vi "stiffnessChartView.vi"(10 "UserEvents in":refnum<class "UserEvents.lvclass">) -> ()   [LabVIEW 2013]
uses:
  UserEvents/UserEvents.lvclass
  UserEvents/UserEvents.lvclass/UserEvents.ctl
  Typedefs/StateSelector.ctl
  Typedefs/M2AADTTypedefs.lvlib
panel:
  out "Stiffness":dbl[unit] min=-888.0 max=888.0 format="%.2f"
  out "Stiffness vs. Move Number":dbl(graph)
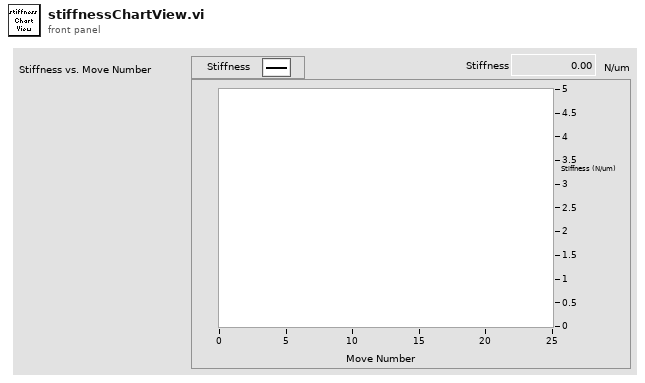
[diagram p1: front panel]
types:
  T1 = typedef "M2AADTTypedefs.lvlib/PubDataEvents.ctl" = cluster{"State":refnum<user-event>, "ErrorCode":refnum<user-event>, "OutputData":refnum<user-event>, "InputData":refnum<user-event>, "ControllerData":refnum<user-event>, "TestStatus":refnum<user-event>, "LogPath":refnum<user-event>, "StiffnessData":refnum<user-event>}
  T2 = cluster{"Event Registration Refnum":refnum<event-registration>, "Event Registration Refnum":refnum<event-registration>}
  T3 = typedef "M2AADTTypedefs.lvlib/StateSelector.ctl" = enum16{"EndingCycleState", "FaultState", "InteractiveMotionState", "MovingToNewForceState", "OffState", "PausingState", "StandbyState", "StoppedState"}
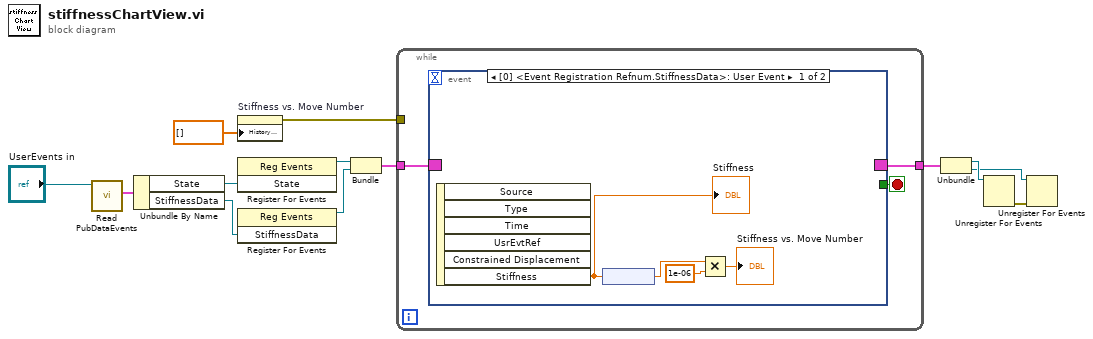
[diagram p0: block diagram]
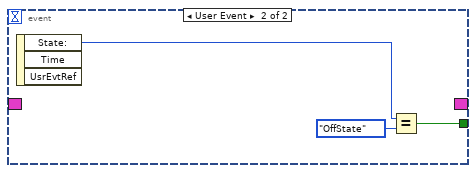
[diagram p2: hidden frame]
diagram:
  n1 = call "Read PubDataEvents.vi"("UserEvents in"="UserEvents in") -> ("PubDataEvents"=w13:T1)  [unwired: 9 in, 1 out]
  n2 = Unbundle By Name(w13) -> ("State"=w12:refnum<user-event>, "StiffnessData"=w3:refnum<user-event>)
  n3 = property on="Stiffness vs. Move Number" class="WFChart (strict)"("History Data"=dbl[] []) -> (error out=w4:errorcluster)  [unwired: 2 in, 1 out]
  n4 = register-events(w12) -> (reference out=w11:refnum<event-registration>)  [unwired: 2 in, 1 out]
  n5 = register-events(w3) -> (reference out=w2:refnum<event-registration>)  [unwired: 2 in, 1 out]
  n6 = Bundle("Event Registration Refnum"=w11, "Event Registration Refnum"=w2) -> (w9:T2)  [unwired: 1 in]
  n7 = while {
    tunnel: w9 -> [w16]
    tunnel: [w14] -> w8
    tunnel: w4 -> [_]
    stop <- w15 stop-if-true
    n8 = event shown="[0] <Event Registration Refnum.StiffnessData>: User Event" {
      selector: w16 -> [_ _]
      dyn-events: [_ _] -> w14
      timeout: _ -> [_ _]
      tunnel: [_ w22] -> w15
      event User Event {
        n9 = event-data() -> ("Stiffness"=w17:dbl[unit])  [unwired: 1 in, 5 out]
        "Stiffness" <- w17
        n10 = node(w17) -> (w20:dbl)
        n11 = Multiply(x=w20, y=1e-06) -> (x*y=→"Stiffness vs. Move Number":dbl)
      }
      event User Event {
        n12 = event-data() -> ("State:"=w21:T3)  [unwired: 1 in, 2 out]
        n13 = Equal?(x=w21, y=StateSelector."OffState" ("State:")) -> (x = y?=w22:bool)
      }
    }
  }
  n14 = Unbundle(w8) -> ("Event Registration Refnum"=w7:refnum<event-registration>, "Event Registration Refnum"=w6:refnum<event-registration>)
  n15 = Unregister For Events(event registration refnum=w7) -> (error out=w5:errorcluster)  [unwired: 1 in]
  n16 = Unregister For Events(event registration refnum=w6, error in=w5) -> ()  [unwired: 1 out]
